vi "03 Charts.vi"() -> ()   [LabVIEW 2019]
panel:
  in  "stop":bool
  out "Waveform Chart":dbl(graph)
  in  "Slide":dbl(slide)=5.204081632653061 scale=0.0..10.0
  # "Hit the Run arrow and see the Chart change as you change the value of the Slide\n\nHit the STOP button to stop"
  # "Hit Cmd E to see the diagram (code)"
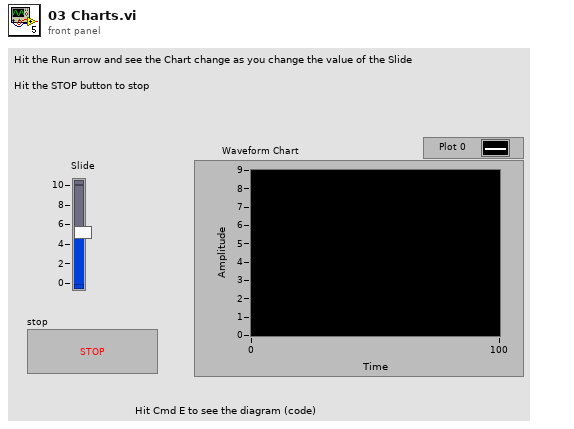
[diagram p1: front panel]
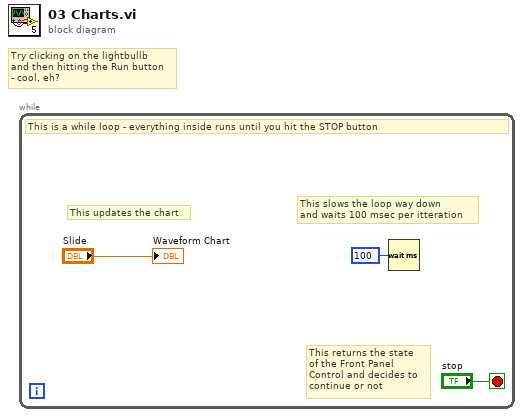
[diagram p0: block diagram]
diagram:
  # "Try clicking on the lightbullb\nand then hitting the Run button\n- cool, eh?"
  n1 = while {
    stop <- "stop" stop-if-true
    # "This returns the state\nof the Front Panel \nControl and decides to\ncontinue or not"
    # "This slows the loop way down \nand waits 100 msec per itteration"
    # "This updates the chart"
    # "This is a while loop - everything inside runs until you hit the STOP button"
    n2 = Wait (ms)(milliseconds to wait=u32 100) -> ()  [unwired: 1 out]
    "Waveform Chart" <- "Slide"
  }
